vi "LCC Read Status.vi"(8 "error in (no error)":errorcluster caption="Fehler (Eingang, kein Fehler)", 11 "Channel Handle":i64) -> (0 "error out":errorcluster caption="Fehler (Ausgang)", 3 "Statusword":u32)   [LabVIEW 2021, in "labbCAN_Controller_API.lvlib"]
doc: "LCC_Func long LCC_CALL LCC_ReadStatus(dev_hdl ChanHdl, unsigned long *pdwStatus);"
uses:
  labbCAN_Controller_API.lvlib
  labbCAN_Controller_API.dll
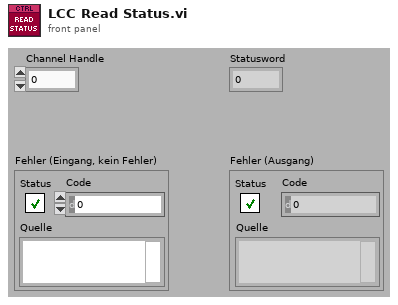
[diagram p1: front panel]
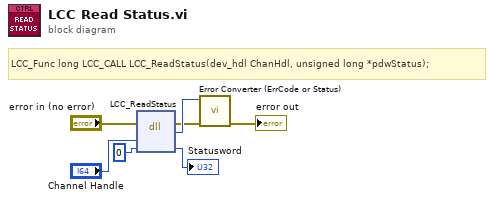
[diagram p0: block diagram]
diagram:
  # "LCC_Func long LCC_CALL LCC_ReadStatus(dev_hdl ChanHdl, unsigned long *pdwStatus);"
  n1 = dll-call lib="C:/Users/olaja/AppData/Local/CETONI_SDK/labbCAN_Controller_API.*" fn="LCC_ReadStatus"(error in="error in (no error)", "ChanHdl"="Channel Handle", "pdwStatus"=u32 0) -> (error out=w2:errorcluster, "Rückgabetyp"=w3:i32, "pdwStatus"=→"Statusword":u32)  [unwired: 3 in, 1 out]
  n2 = call "Error Converter (ErrCode or Status).vi"("error in (no error)"=w2, "error code"=w3) -> ("error out"=→"error out":errorcluster)  [unwired: 9 in]
